vi "saveUSB650backup.vi"(4 "position notes":string, 5 "Integration Time":dbl, 6 "(units)":string, 7 "wavelengths":dbl[](array[numeric]), 8 "Position of Lens":dbl, 9 "time":dbl[](array[numeric]), 10 "Counts":dbl[][](array[numeric]), 11 "appended path":path) -> ()   [LabVIEW 2011]
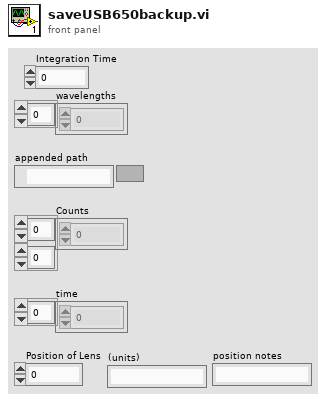
[diagram p1: front panel]
types:
  T1 = enum16{"open", "replace", "create", "open or create", "replace or create", "replace or create with confirmation"}
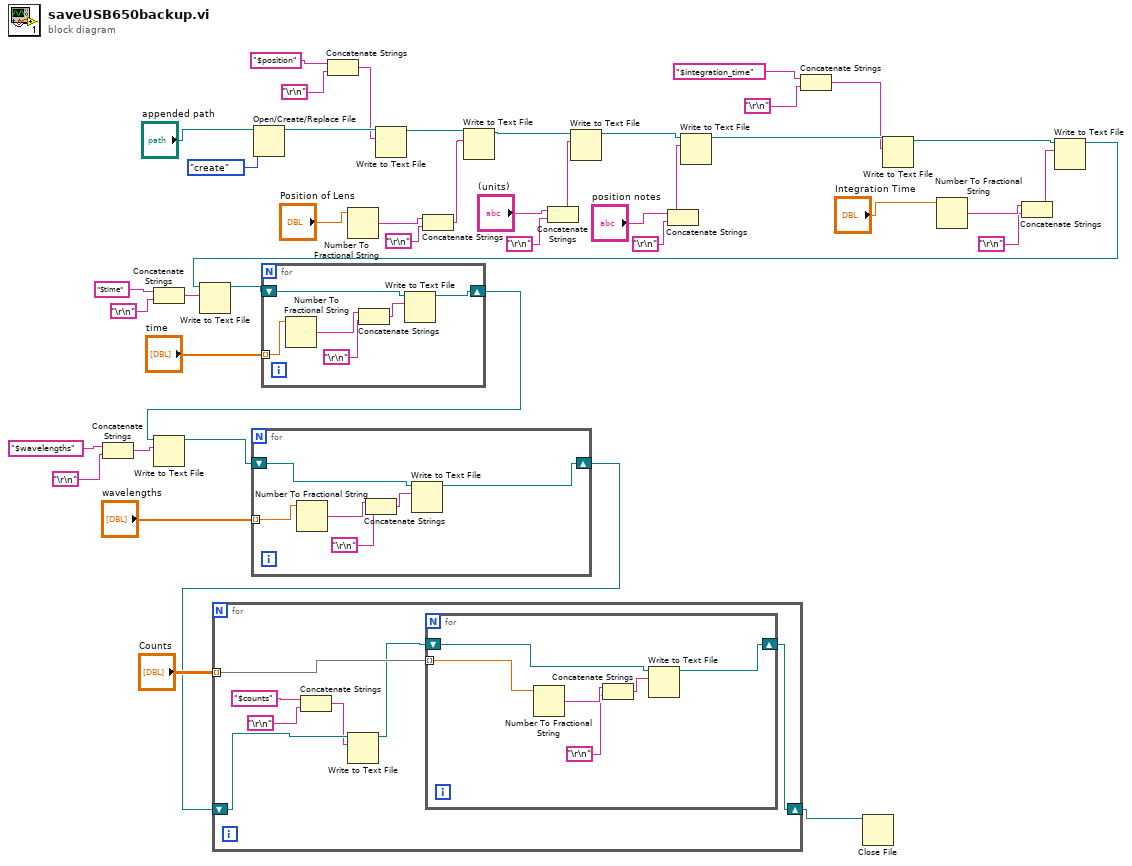
[diagram p0: block diagram]
diagram:
  n1 = Concatenate Strings("$wavelengths" ("text"), "\r\n") -> (w16:string)
  n2 = Concatenate Strings("$time" ("text"), "\r\n") -> (w19:string)
  n3 = Open/Create/Replace File(file path (use dialog)="appended path", operation (0:open)=T1."create") -> (refnum out=w41:refnum<file>)  [unwired: 4 in, 2 out]
  n4 = Concatenate Strings("$position" ("text"), "\r\n") -> (w11:string)
  n5 = Number To Fractional String(number="Position of Lens") -> (F-format string=w26:string)  [unwired: 3 in]
  n6 = Write to Text File(file (use dialog)=w41, text=w11) -> (refnum out=w39:refnum<file>)  [unwired: 2 in, 2 out]
  n7 = Concatenate Strings(w26, "\r\n") -> (w40:string)
  n8 = Write to Text File(file (use dialog)=w39, text=w40) -> (refnum out=w38:refnum<file>)  [unwired: 2 in, 2 out]
  n9 = Concatenate Strings("(units)", "\r\n") -> (w36:string)
  n10 = Write to Text File(file (use dialog)=w38, text=w36) -> (refnum out=w34:refnum<file>)  [unwired: 2 in, 2 out]
  n11 = Concatenate Strings("position notes", "\r\n") -> (w33:string)
  n12 = Write to Text File(file (use dialog)=w34, text=w33) -> (refnum out=w8:refnum<file>)  [unwired: 2 in, 2 out]
  n13 = Concatenate Strings("$integration_time", "\r\n") -> (w7:string)
  n14 = Write to Text File(file (use dialog)=w8, text=w7) -> (refnum out=w3:refnum<file>)  [unwired: 2 in, 2 out]
  n15 = Number To Fractional String(number="Integration Time") -> (F-format string=w5:string)  [unwired: 3 in]
  n16 = Concatenate Strings(w5, "\r\n") -> (w2:string)
  n17 = Write to Text File(file (use dialog)=w3, text=w2) -> (refnum out=w1:refnum<file>)  [unwired: 2 in, 2 out]
  n18 = Write to Text File(file (use dialog)=w1, text=w19) -> (refnum out=w31:refnum<file>)  [unwired: 2 in, 2 out]
  n19 = for {
    tunnel: "time" -> [w46] mode=indexing
    shift-right: [w48] -> w30
    shift-left: w31 -> [w47]
    n20 = Number To Fractional String(number=w46) -> (F-format string=w45:string)  [unwired: 3 in]
    n21 = Concatenate Strings(w45, "\r\n") -> (w49:string)
    n22 = Write to Text File(file (use dialog)=w47, text=w49) -> (refnum out=w48:refnum<file>)  [unwired: 2 in, 2 out]
  }
  n23 = Write to Text File(file (use dialog)=w30, text=w16) -> (refnum out=w29:refnum<file>)  [unwired: 2 in, 2 out]
  n24 = for {
    shift-right: [w53] -> w24
    shift-left: w29 -> [w54]
    tunnel: "wavelengths" -> [w52] mode=indexing
    n25 = Number To Fractional String(number=w52) -> (F-format string=w51:string)  [unwired: 3 in]
    n26 = Concatenate Strings(w51, "\r\n") -> (w55:string)
    n27 = Write to Text File(file (use dialog)=w54, text=w55) -> (refnum out=w53:refnum<file>)  [unwired: 2 in, 2 out]
  }
  n28 = for {
    tunnel: "Counts" -> [w62] mode=indexing
    shift-right: [w59] -> w23
    shift-left: w24 -> [w61]
    n29 = Concatenate Strings("$counts" ("text"), "\r\n") -> (w56:string)
    n30 = Write to Text File(file (use dialog)=w61, text=w56) -> (refnum out=w60:refnum<file>)  [unwired: 2 in, 2 out]
    n31 = for {
      tunnel: w62 -> [w65] mode=indexing
      shift-right: [w64] -> w59
      shift-left: w60 -> [w66]
      n32 = Number To Fractional String(number=w65) -> (F-format string=w67:string)  [unwired: 3 in]
      n33 = Concatenate Strings(w67, "\r\n") -> (w68:string)
      n34 = Write to Text File(file (use dialog)=w66, text=w68) -> (refnum out=w64:refnum<file>)  [unwired: 2 in, 2 out]
    }
  }
  n35 = Close File(refnum=w23) -> ()  [unwired: 1 in, 2 out]
